vi "act-0021-2-cor.vi"() -> ()   [LabVIEW 2010]
uses:
  support/c_pi_wilson.ctl
  support/c_pi_penalite.ctl
  support/c_pi_stock.ctl
  support/c_pi_stock_O-N.ctl
  support/lv_07.lvlib
panel:
  out "Stockage (sortie)":T1
  in  "Pénalité (e)":T3
  in  "Pièce e":T4
  out "error out":errorcluster caption="err out"
  in  "err in":errorcluster
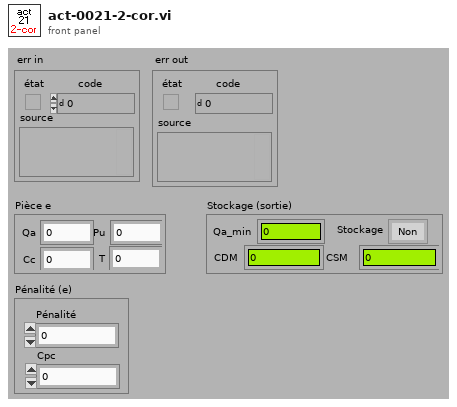
[diagram p1: front panel]
types:
  T1 = typedef "lv_07.lvlib/c_pi_stock.ctl" = cluster{"Qa_min":dbl, "CDM":dbl, "CSM":dbl, "Stockage":T2}
  T2 = typedef "lv_07.lvlib/c_pi_stock_O-N.ctl" = enum16{"Non", "Oui"}
  T3 = typedef "lv_07.lvlib/c_pi_penalite.ctl" = cluster{"Pénalité":dbl, "Cpc":dbl}
  T4 = typedef "lv_07.lvlib/c_pi_wilson.ctl" = cluster{"T":dbl, "Pu":dbl, "Qa":dbl, "Cc":dbl}
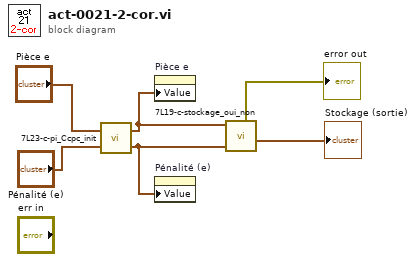
[diagram p0: block diagram]
diagram:
  n1 = call "7L23-c-pi_Ccpc_init.vi"("Pénalité (e)"="Pénalité (e)", "Pièce e"="Pièce e") -> ("Pénalité (s)"=w3:T3, "Pièce s"=w4:T4)
  n2 = property on="Pièce e" class="Clust (strict)"("Value"=w4) -> ()  [unwired: 2 in, 2 out]
  n3 = property on="Pénalité (e)" class="Clust (strict)"("Value"=w3) -> ()  [unwired: 2 in, 2 out]
  n4 = call "7L19-c-stockage_oui_non.vi"("Pénalité (e)"=w3, "Pièce (e)"=w4) -> ("Stockage (sortie)"=→"Stockage (sortie)":T1, "err out"=→"error out":errorcluster)  [unwired: 4 in, 2 out]
